vi "Generate Scan Values.vi"(0 "Number of Steps":i32, 7 "Center Value":dbl=7.0, 11 "Step Size":dbl) -> (8 "Scan Values":dbl[](array[numeric]))   [LabVIEW 2020]
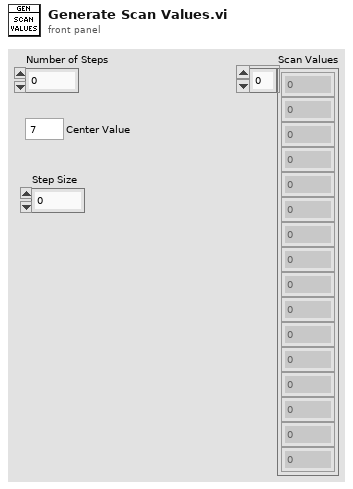
[diagram p1: front panel]
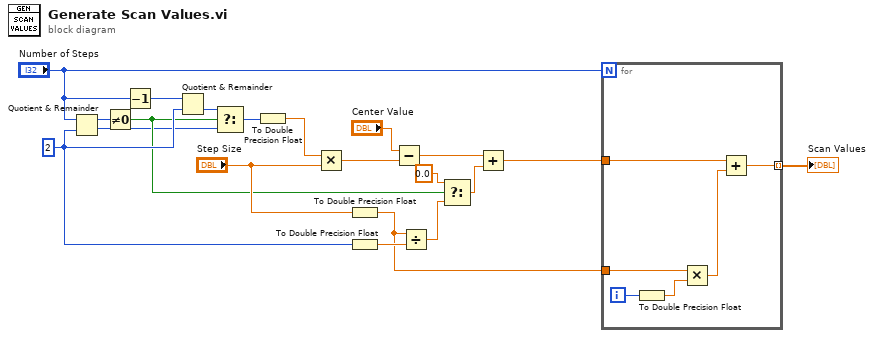
[diagram p0: block diagram]
diagram:
  w18 = 2 ("y")
  n1 = Quotient & Remainder(x="Number of Steps", y=w18) -> (x-y*floor(x/y)=w7:i32, floor(x/y)=w10:i32)
  n2 = Not Equal To 0?(x=w7) -> (x != 0?=w17:bool)
  n3 = Decrement(x="Number of Steps") -> (x-1=w8:i32)
  n4 = Quotient & Remainder(x=w8, y=w18) -> (floor(x/y)=w9:i32)  [unwired: 1 out]
  n5 = Select(t=w9, s=w17, f=w10) -> (s? t:f=w11:i32)
  n6 = To Double Precision Float(number=w11) -> (double precision float=w2:dbl)
  n7 = Multiply(x=w2, y="Step Size") -> (x*y=w1:dbl)
  n8 = To Double Precision Float(number="Step Size") -> (double precision float=w4:dbl)
  n9 = To Double Precision Float(number=w18) -> (double precision float=w19:dbl)
  n10 = Subtract(x="Center Value", y=w1) -> (x-y=w13:dbl)
  n11 = Divide(x=w4, y=w19) -> (x/y=w14:dbl)
  n12 = Select(t=0.0, s=w17, f=w14) -> (s? t:f=w15:dbl)
  n13 = Add(x=w13, y=w15) -> (x+y=w5:dbl)
  n14 = for {
    N: "Number of Steps" -> [_]
    tunnel: w5 -> [w26]
    tunnel: w4 -> [w24]
    tunnel: [w21] -> w3 mode=indexing
    i -> [w25]
    n15 = To Double Precision Float(number=w25) -> (double precision float=w23:dbl)
    n16 = Multiply(x=w24, y=w23) -> (x*y=w22:dbl)
    n17 = Add(x=w26, y=w22) -> (x+y=w21:dbl)
  }
  "Scan Values" <- w3
